vi "Initialize Thor WP.vi"(3 "error in (no error)":errorcluster, 5 "input Kcube refnum cluster":T1) -> (0 "error out":errorcluster, 2 "output Kcube cluster":T1)   [LabVIEW 2015]
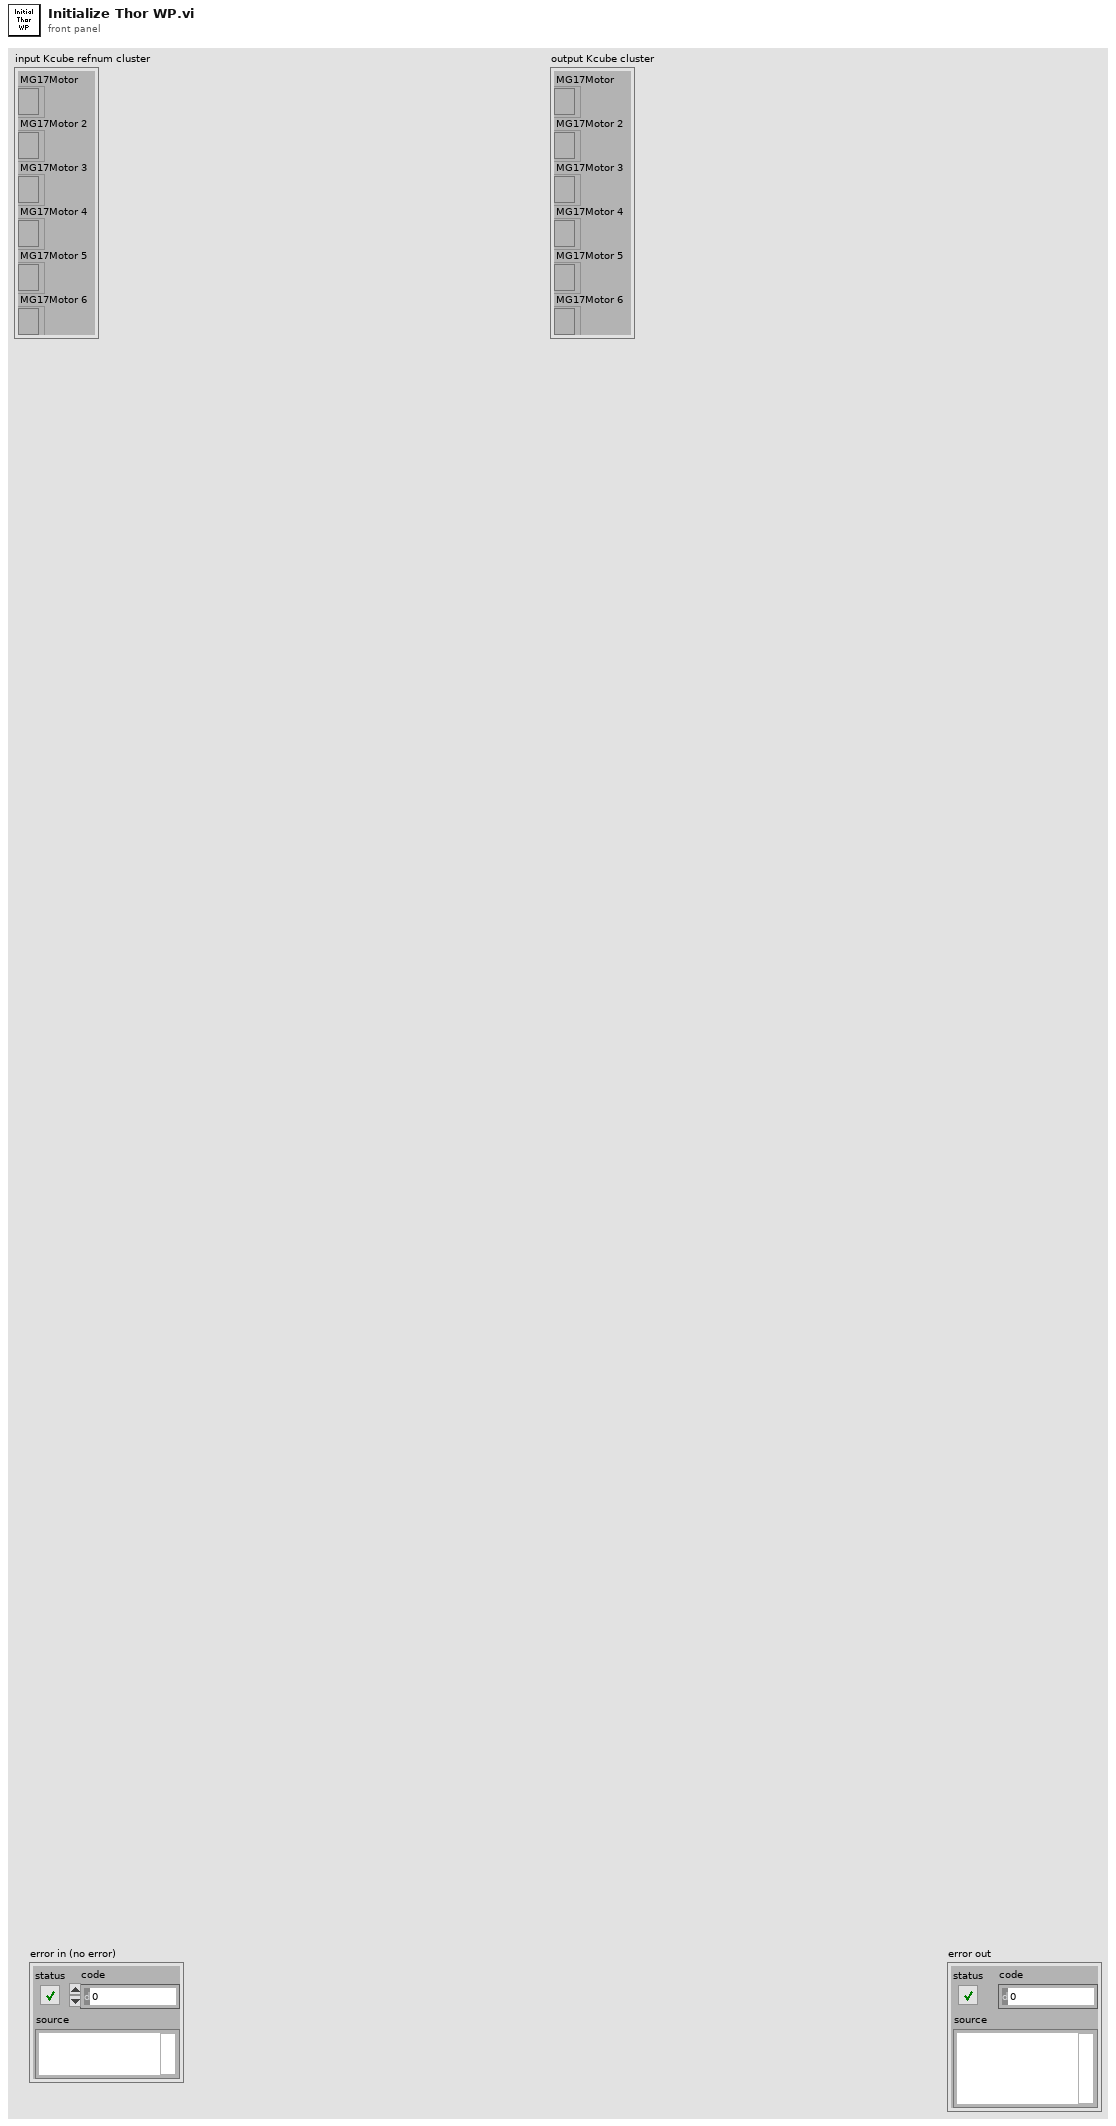
[diagram p1: front panel]
types:
  T1 = cluster{"MG17Motor":refnum<k7>, "MG17Motor 2":refnum<k7>, "MG17Motor 3":refnum<k7>, "MG17Motor 4":refnum<k7>, "MG17Motor 5":refnum<k7>, "MG17Motor 6":refnum<k7>}
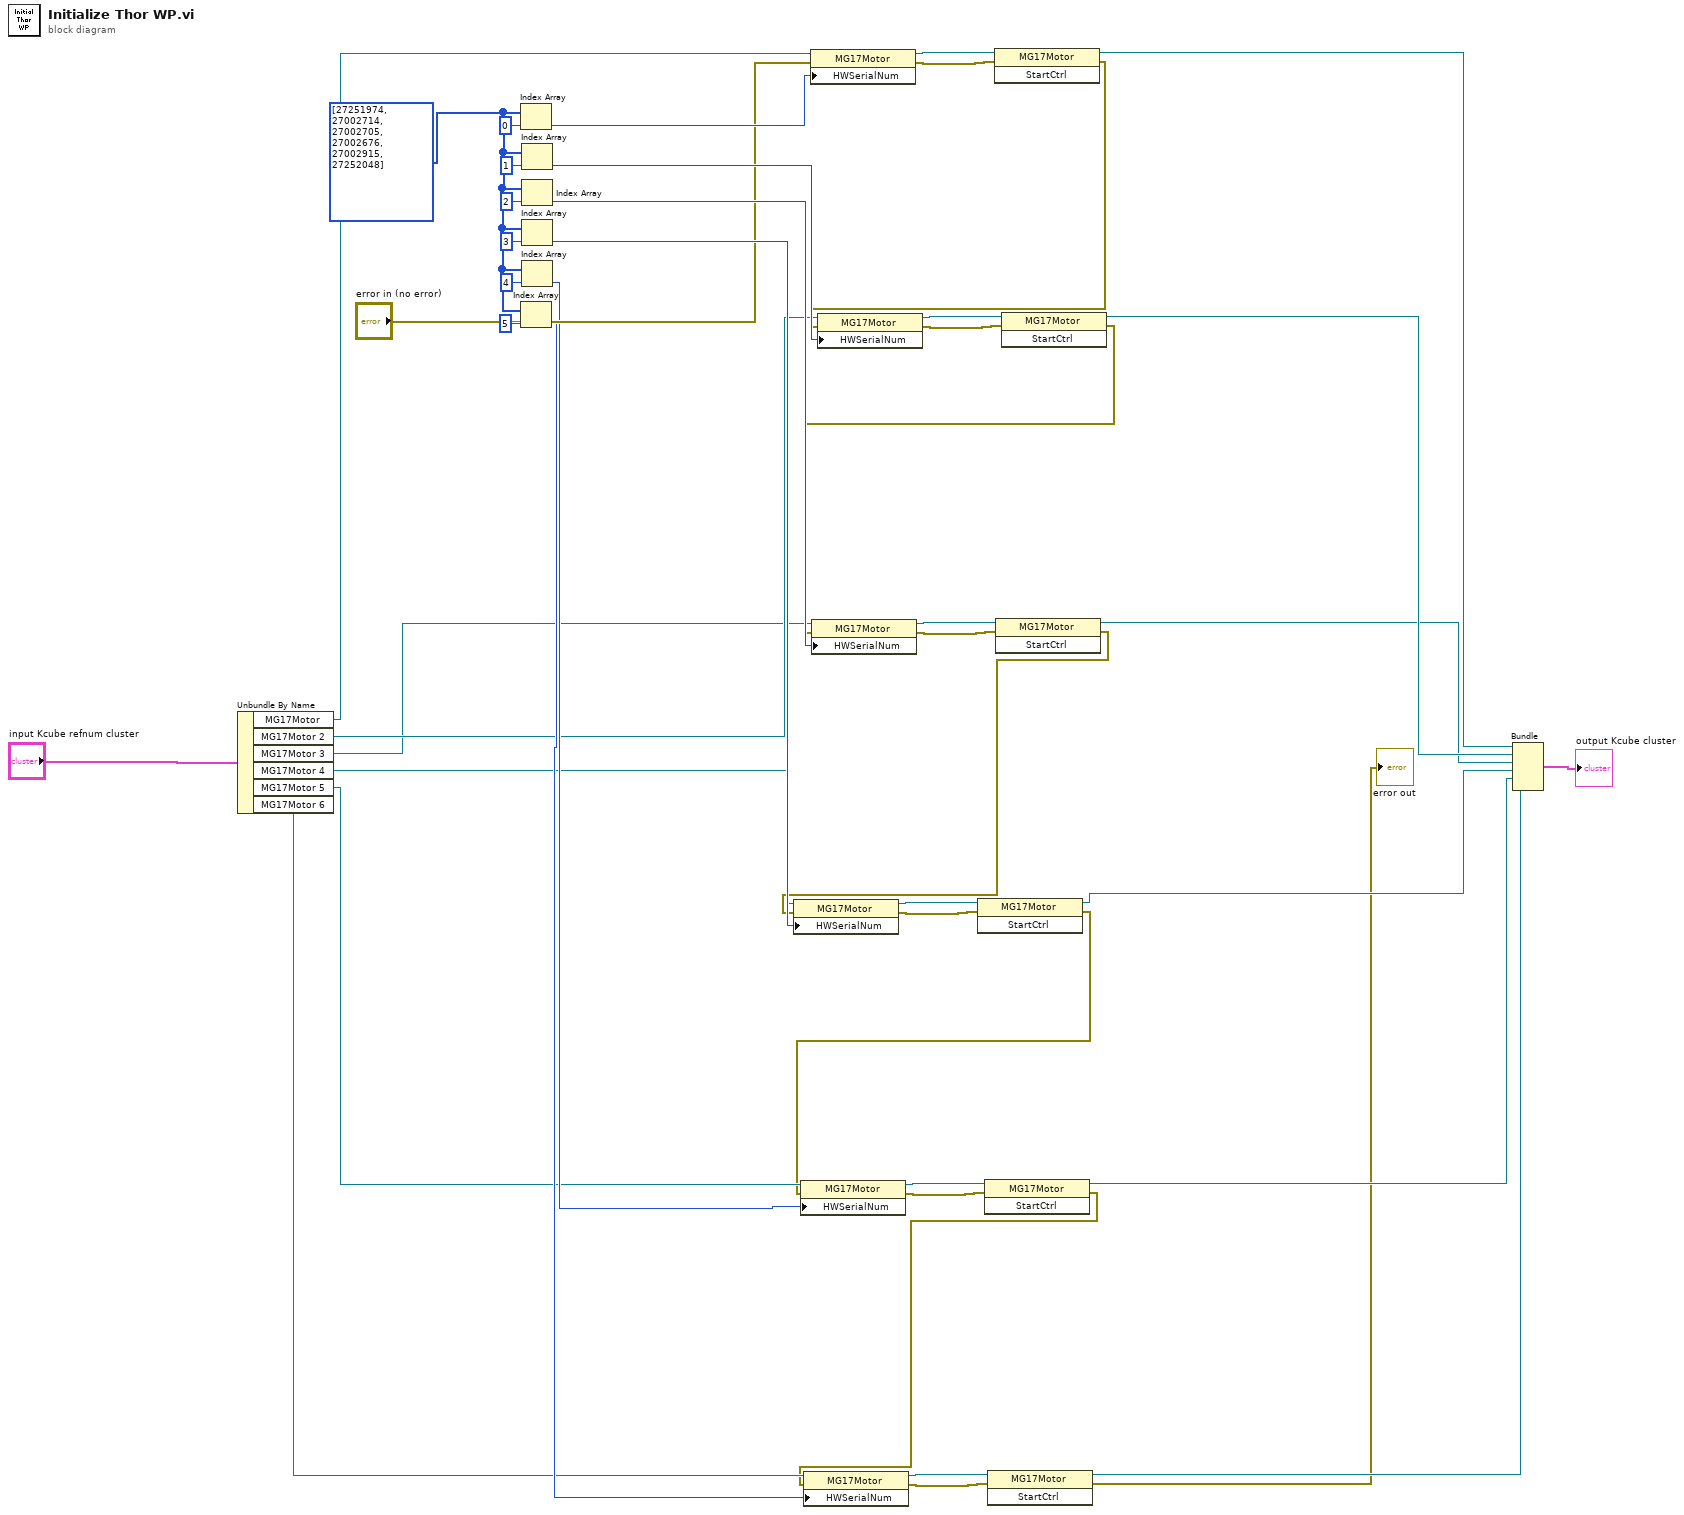
[diagram p0: block diagram]
diagram:
  w41 = i32[] [27251974, 27002714, 27002705, 27002676, 27002915, 27252048]
  n1 = Unbundle By Name("input Kcube refnum cluster") -> ("MG17Motor"=w39:refnum<k7>, "MG17Motor 2"=w19:refnum<k7>, "MG17Motor 3"=w18:refnum<k7>, "MG17Motor 4"=w17:refnum<k7>, "MG17Motor 5"=w16:refnum<k7>, "MG17Motor 6"=w15:refnum<k7>)
  n2 = Index Array(array=w41, index=0) -> (element=w38:i32)
  n3 = Index Array(array=w41, index=5) -> (element=w20:i32)
  n4 = Index Array(array=w41, index=1) -> (element=w25:i32)
  n5 = Index Array(array=w41, index=2) -> (element=w24:i32)
  n6 = Index Array(array=w41, index=3) -> (element=w23:i32)
  n7 = Index Array(array=w41, index=4) -> (element=w21:i32)
  n8 = property class="MG17Motor"(reference=w39, error in="error in (no error)", "HWSerialNum"=w38) -> (reference out=w37:refnum<k7>, error out=w36:errorcluster)
  n9 = invoke class="MG17Motor" method="StartCtrl"(reference=w37, error in=w36) -> (reference out=w14:refnum<k7>, error out=w7:errorcluster)  [unwired: 1 in, 1 out]
  n10 = property class="MG17Motor"(reference=w19, error in=w7, "HWSerialNum"=w25) -> (reference out=w35:refnum<k7>, error out=w34:errorcluster)
  n11 = invoke class="MG17Motor" method="StartCtrl"(reference=w35, error in=w34) -> (reference out=w13:refnum<k7>, error out=w6:errorcluster)  [unwired: 1 in, 1 out]
  n12 = property class="MG17Motor"(reference=w18, error in=w6, "HWSerialNum"=w24) -> (reference out=w33:refnum<k7>, error out=w32:errorcluster)
  n13 = invoke class="MG17Motor" method="StartCtrl"(reference=w33, error in=w32) -> (reference out=w12:refnum<k7>, error out=w5:errorcluster)  [unwired: 1 in, 1 out]
  n14 = property class="MG17Motor"(reference=w17, error in=w5, "HWSerialNum"=w23) -> (reference out=w31:refnum<k7>, error out=w30:errorcluster)
  n15 = invoke class="MG17Motor" method="StartCtrl"(reference=w31, error in=w30) -> (reference out=w11:refnum<k7>, error out=w4:errorcluster)  [unwired: 1 in, 1 out]
  n16 = property class="MG17Motor"(reference=w16, error in=w4, "HWSerialNum"=w21) -> (reference out=w29:refnum<k7>, error out=w28:errorcluster)
  n17 = invoke class="MG17Motor" method="StartCtrl"(reference=w29, error in=w28) -> (reference out=w10:refnum<k7>, error out=w3:errorcluster)  [unwired: 1 in, 1 out]
  n18 = property class="MG17Motor"(reference=w15, error in=w3, "HWSerialNum"=w20) -> (reference out=w27:refnum<k7>, error out=w26:errorcluster)
  n19 = invoke class="MG17Motor" method="StartCtrl"(reference=w27, error in=w26) -> (reference out=w9:refnum<k7>, error out=→"error out":errorcluster)  [unwired: 1 in, 1 out]
  n20 = Bundle("MG17Motor"=w14, "MG17Motor 2"=w13, "MG17Motor 3"=w12, "MG17Motor 4"=w11, "MG17Motor 5"=w10, "MG17Motor 6"=w9) -> (→"output Kcube cluster":T1)  [unwired: 1 in]
